vi "get_config_cluster.vi"(8 "error in (no error)":errorcluster, 11 "LightSourceMH110125Tsunami in":refnum<class "LightSourceMH110125Tsunami.lvclass">) -> (0 "error out":errorcluster, 2 "config cluster (variant)":variant, 3 "LightSourceMH110125Tsunami out":refnum<class "LightSourceMH110125Tsunami.lvclass">)   [LabVIEW 2010, in "LightSourceMH110125Tsunami.lvclass"]
uses:
  LightSourceMH110125Tsunami.lvclass
  LightSourceMH110125Tsunami.lvclass/LightSourceMH110125Tsunami.ctl
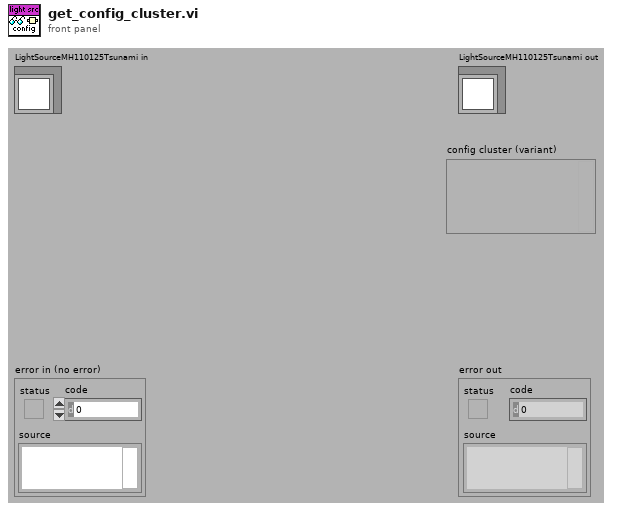
[diagram p1: front panel]
types:
  T1 = typedef "LightSourceMH110125Tsunami.lvclass/config_data_cluster.ctl" = cluster{"hardware settings":cluster{"comm port":string, "switch laser on?":bool, "open shutter?":bool, "max power":dbl[unit], "delay before read (ms)":u32, "flow control":u16, "stop bits":u16, "data bits":u16, "baud rate":u32, "parity (0:none)":enum16{"None", "Odd", "Even", "Mark", "Space"}}, "OME":cluster{"LSID":T2, "manufacturer specification":T3, "frequency multiplication":dbl, "tuneable?":bool, "repetition rate":dbl[unit], "pump laser configuration":string, "laser medium":T4, "pulse":T5, "type":T6}}
  T2 = typedef "LSID_cluster.ctl" = cluster{"identifier":string, "revision":i32}
  T3 = typedef "GenericComponent.lvclass/manufacturer_specification_cluster.ctl" = cluster{"manufacturer":string, "model":string, "serial number":string, "lot number":string}
  T4 = typedef "LightSourceMH110125Tsunami.lvclass/laser_medium_enum.ctl" = enum16{"Cu", "Ag", "ArFl", "ArCl", "KrFl", "XeFl", "XeCl", "XeBr", "N", "Ar", "Kr", "Xe", "HeNe", "HeCd", "CO", "CO2", "H2O", "HFl", "NdGlass", "NdYAG", "ErGlass", "ErYAG", "HoYLF", "HoYAG", "Ruby", "TiSapphire", "Alexandrite", "Rhodamine6G", "CoumarineC30", "GaAs", "GaAlAs", "EMinus", "Unknown"}
  T5 = typedef "LightSourceMH110125Tsunami.lvclass/pulse_enum.ctl" = enum16{"CW", "Single", "QSwitched", "Repetitive", "ModeLocked"}
  T6 = typedef "LightSourceMH110125Tsunami.lvclass/type_enum.ctl" = enum16{"Excimer", "Gas", "MetalVapor", "SolidState", "Dye", "Semiconductor", "FreeElectron", "Unknown"}
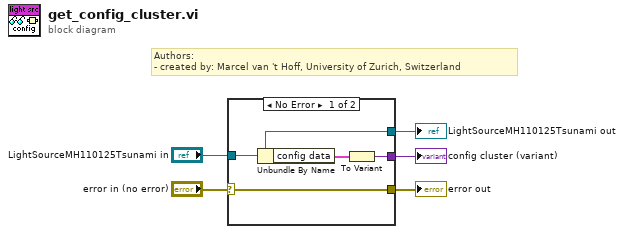
[diagram p0: block diagram]
diagram:
  # "Authors: \n- created by: Marcel van 't Hoff, University of Zurich, Switzerland"
  n1 = case shown="No Error" "error in (no error)" {
    selector: "error in (no error)" -> [w6 w10]
    tunnel: "LightSourceMH110125Tsunami in" -> [w8 w11]
    tunnel: [w8 w11] -> w2
    tunnel: [w7 _] -> w3
    tunnel: [w6 w10] -> w1
    frame No Error {
      n2 = Unbundle By Name(w8) -> ("config data"=w9:T1)
      n3 = To Variant(anything=w9) -> (Variant=w7:variant)
    }
    frame Error {
    }
  }
  "error out" <- w1
  "LightSourceMH110125Tsunami out" <- w2
  "config cluster (variant)" <- w3
